vi "IMIC_IsInit.vi"(0 "handle":i32) -> (1 "output param":T1(ring), 2 "handle out":i32, 3 "bool":i8)   [LabVIEW 8.6]
uses:
  Program Files/colibri/Drivers/TILLPhotonics/tillimic.dll
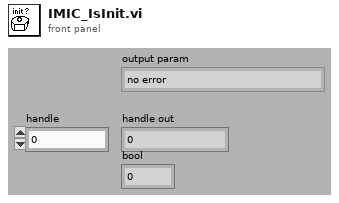
[diagram p1: front panel]
types:
  T1 = enum16{"no error", "missing axis", "missing Z axis", "missing Filter", "iMic not initialized", "no property", "wrong handle", "protocol not finished", "user parameter to long (>32 bits)", "no user parameter handle", "failed to open comport", "failed to initialize"}
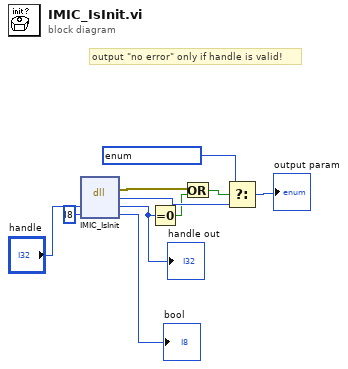
[diagram p0: block diagram]
diagram:
  # "output \"no error\" only if handle is valid!"
  n1 = dll-call lib="C:/colibri-laserscanning/Drivers/TILLPhotonics/tillimic.dll" fn="IMIC_IsInit"("handle"="handle", "bool"=i8 ?) -> (error out=w4:errorcluster, w7:i32, "handle"=w3:i32, "bool"=→"bool":i8)  [unwired: 3 in, 1 out]
  "handle out" <- w3
  n2 = Equal To 0?(x=w3) -> (x = 0?=w2:bool)
  n3 = Or(x=w4, y=w2) -> (x .or. y?=w1:bool)
  n4 = Select(t=T1 ? ("output param"), s=w1, f=w7) -> (s? t:f=→"output param":i32)
